vi "dataUnpackDBL.vi"(8 "errorIn":errorcluster, 11 "data":variant) -> (0 "errorOut":errorcluster, 3 "DBL":dbl)   [LabVIEW 2017]
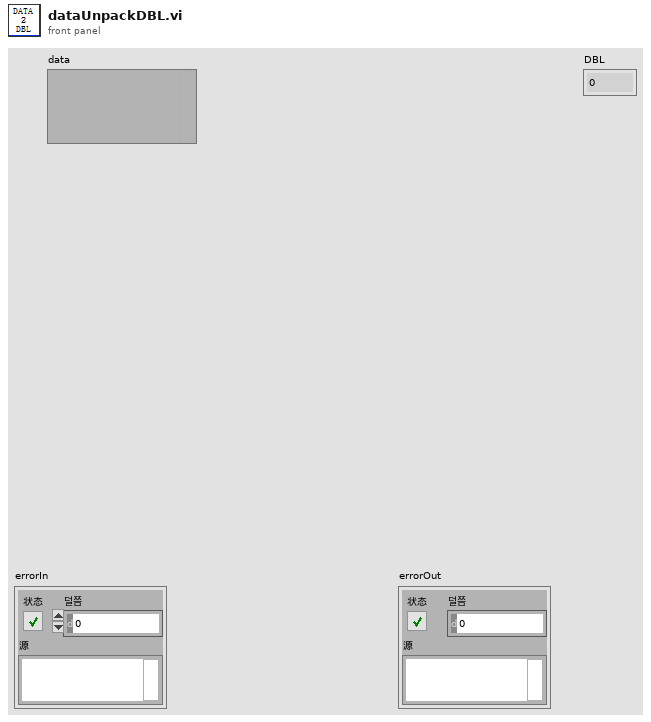
[diagram p1: front panel]
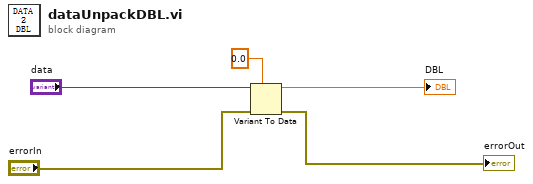
[diagram p0: block diagram]
diagram:
  n1 = Variant To Data(error in="errorIn", type=0.0, Variant="data") -> (data=→"DBL":dbl, error out=→"errorOut":errorcluster)
